vi "Path.vi"(8 "error in":errorcluster) -> (0 "error out":errorcluster, 2 "Cancelled":bool caption="cancelled", 3 "Selected Path":path caption="selected path")   [LabVIEW 2023, in "Registration.lvclass"]
uses:
  Registration.lvclass
  Registration.lvclass/Registration.ctl
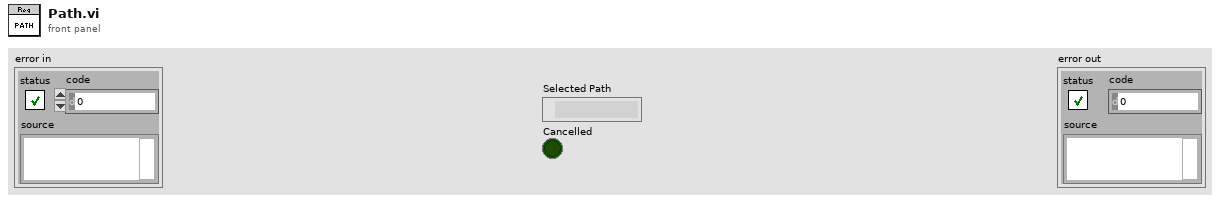
[diagram p1: front panel]
types:
  T1 = enum16{"open", "replace", "create", "open or create", "replace or create", "replace or create with confirmation"}
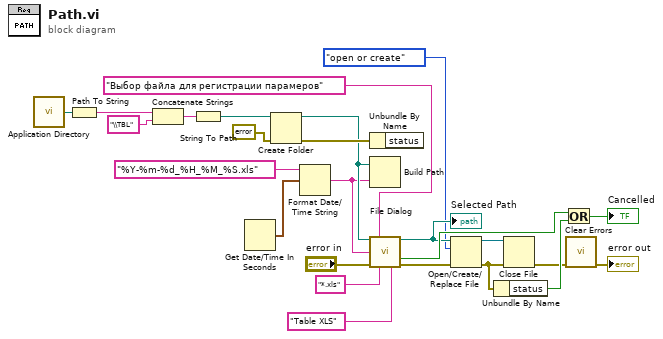
[diagram p0: block diagram]
diagram:
  n1 = call <vilib>:"Application Directory.vi"() -> ("Application Directory"=w21:path)
  n2 = Path To String(path=w21) -> (string=w22:string)
  n3 = Concatenate Strings(w22, "\\TBL" ("string")) -> (w24:string)
  n4 = String To Path(string=w24) -> (path=w23:path)
  n5 = Get Date/Time In Seconds() -> (seconds since 1Jan1904=w20:timestamp)
  n6 = Create Folder(path (use dialog)=w23, error in=errorcluster {"status"=FALSE, "code"=0, "source"=""} ("error in (no error)")) -> (created path=w13:path, error out=w25:errorcluster)  [unwired: 1 in, 1 out]
  n7 = Format Date/Time String(time format string (%c)="%Y-%m-%d_%H_%M_%S.xls", seconds (now)=w20) -> (date/time string=w12:string)  [unwired: 1 in]
  n8 = Unbundle By Name(w25) -> ()  [unwired: 1 out]
  n9 = Build Path(base path=w13, name or relative path=w12) -> ()  [unwired: 1 out]
  n10 = call "File Dialog"("start path"=w13, "prompt"="Выбор файла для регистрации парамеров", "default name"=w12, "error in"="error in", "pattern (all files)"="*.xls", "pattern label"="Table XLS") -> ("selected path"=w7:path, "cancelled"=w11:bool, "error out"=w5:errorcluster)  [unwired: 6 in, 1 out]
  "Selected Path" <- w7
  n11 = Open/Create/Replace File(file path (use dialog)=w7, error in=w5, operation (0:open)=T1."open or create") -> (refnum out=w4:refnum<file>, error out=w3:errorcluster)  [unwired: 3 in, 1 out]
  n12 = Unbundle By Name(w3) -> ("status"=w8:bool)
  n13 = Close File(refnum=w4, error in=w3) -> (error out=w2:errorcluster)  [unwired: 1 out]
  n14 = Or(x=w11, y=w8) -> (x .or. y?=→"Cancelled":bool)
  n15 = call <vilib>:"Clear Errors.vi"("error in (no error)"=w2) -> ("error out"=→"error out":errorcluster)  [unwired: 5 in, 1 out]
